vi "DSF.Engine.BuilderManager.Launch Builders.vi"(8 "error in (no error)":errorcluster, 10 "Thread Parameters":refnum<class "Thread Parameters.lvclass">, 11 "Builder Manager in":refnum<class "DSF.Engine.BuilderManager.lvclass">) -> (0 "error out":errorcluster, 3 "Builder Manager out":refnum<class "DSF.Engine.BuilderManager.lvclass">)   [LabVIEW 2016, in "DSF.Engine.lvlib" / "DSF.Engine.BuilderManager.lvclass"]
uses:
  DSF.Engine.BuilderManager.lvclass
  Thread Parameters/Thread Parameters.lvclass
  DSF.Engine.BuilderManager.lvclass/DSF.Engine.BuilderManager.ctl
  Builder/DSF.Engine.Builder.lvclass
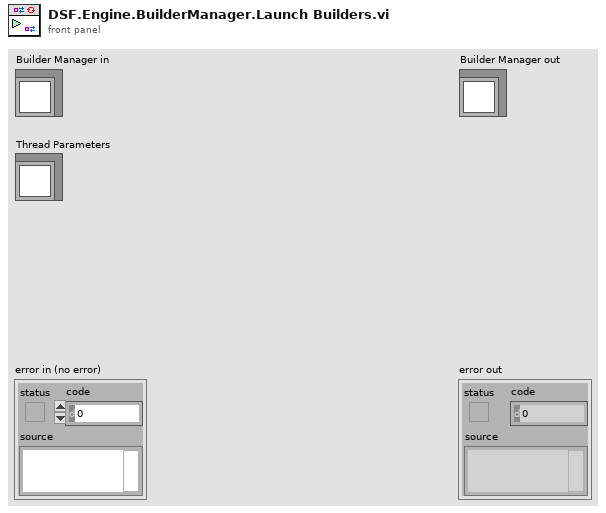
[diagram p1: front panel]
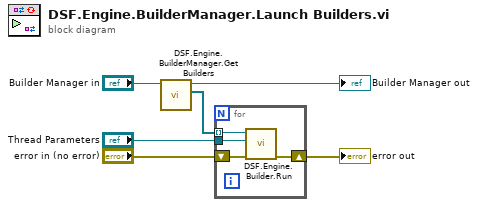
[diagram p0: block diagram]
diagram:
  n1 = call "DSF.Engine.BuilderManager.Get Builders.vi"("Builder Manager in"="Builder Manager in") -> ("Builders"=w2:refnum<class "DSF.Engine.Builder.lvclass">[], "Builder Manager out"=→"Builder Manager out":refnum<class "DSF.Engine.BuilderManager.lvclass">)  [unwired: 9 in]
  n2 = for {
    shift-right: [w9] -> w6
    shift-left: "error in (no error)" -> [w10]
    tunnel: w2 -> [w8] mode=indexing
    tunnel: "Thread Parameters" -> [w7]
    n3 = call "DSF.Engine.Builder.Run.vi"("error in (no error)"=w10, "Thread Parameters"=w7, "Builder in"=w8) -> ("error out"=w9:errorcluster)  [unwired: 6 in, 2 out]
  }
  "error out" <- w6
